vi "gh-cli Version.vi"(8 "error in (no error)":errorcluster, 11 "Git in":refnum<class "Git.lvclass">) -> (0 "error out":errorcluster, 2 "version":string, 3 "Git out":refnum<class "Git.lvclass">)   [LabVIEW 2019, in "Git.lvclass"]
doc: "gh --version: Show gh version \n\nhttps://cli.github.com/manual"
uses:
  Git.lvclass
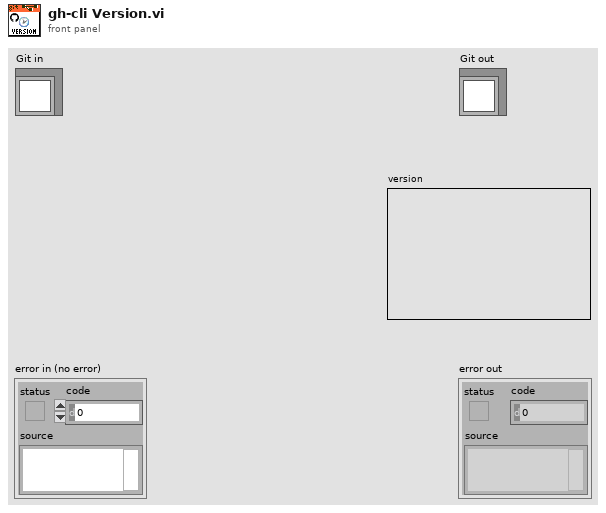
[diagram p1: front panel]
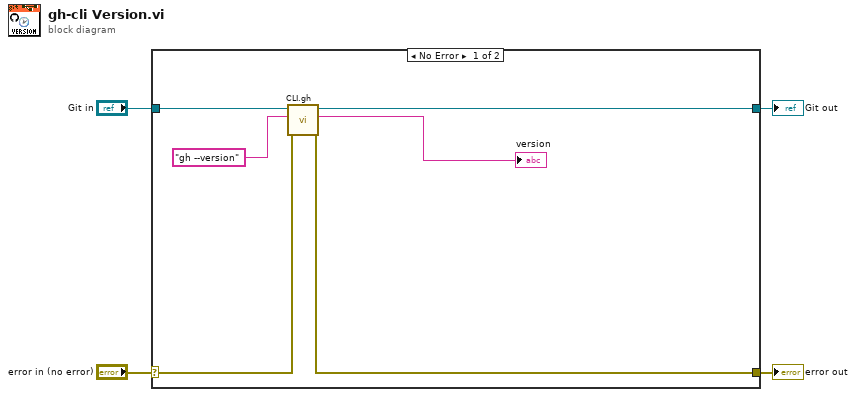
[diagram p0: block diagram]
diagram:
  n1 = case shown="No Error" "error in (no error)" {
    selector: "error in (no error)" -> [w8 w12]
    tunnel: [w7 w12] -> w3
    tunnel: [w9 w11] -> w1
    tunnel: "Git in" -> [w10 w11]
    frame No Error {
      n2 = call "CLI.gh.vi"("error in (no error)"=w8, "Command"="gh --version", "Git in"=w10) -> ("error out"=w7:errorcluster, "standard output"=→"version":string, "Git out"=w9:refnum<class "Git.lvclass">)  [unwired: 4 in, 2 out]
    }
    frame Error {
    }
  }
  "error out" <- w3
  "Git out" <- w1
